vi "Populate File Info.vi"(8 "error in":errorcluster, 11 "UI Actor in":refnum<class "UI Actor.lvclass">) -> (0 "error out":errorcluster, 3 "UI Actor out":refnum<class "UI Actor.lvclass">)   [LabVIEW 2024, in "UI Actor.lvlib" / "UI Actor.lvclass"]
uses:
  UI Actor.lvclass
  Controls/File Info.ctl
  UI Actor.lvclass/UI Actor.ctl
  Core/File Info/File Info.lvclass
  Core/EDS/EDS.lvclass
  <vilib>/Utility/Data Type/NI_Data Type.lvlib
  <userlib>/_OpenG.lib/lvdata/lvdata.llb/openg_variant.lvlib
  <vilib>/JDP Science/JDP Science Common Utilities/JDP Utility.lvlib
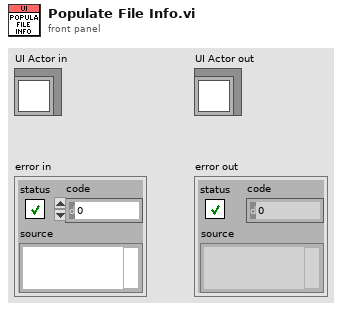
[diagram p1: front panel]
types:
  T1 = typedef "File Info.ctl" = cluster{"FileVersion":u8, "FileRevision":u8, "EDSVersion":string, "Description":string, "CreationDate":string, "CreationTime":string, "CreatedBy":string, "ModificationDate":string, "ModificationTime":string, "ModifiedBy":string}
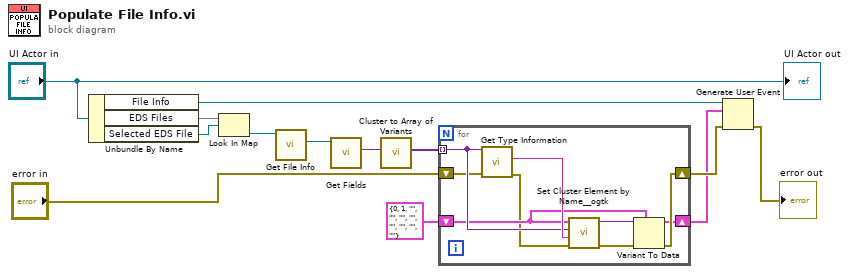
[diagram p0: block diagram]
diagram:
  n1 = Unbundle By Name("UI Actor in") -> ("File Info"=w13:refnum<user-event>, "EDS Files"=w9:map{path, refnum<class "EDS.lvclass">}, "Selected EDS File"=w8:path)
  n2 = Look In Map(map=w9, key=w8) -> (value=w10:refnum<class "EDS.lvclass">)  [unwired: 1 in, 1 out]
  n3 = call "Get File Info.vi"("EDS in"=w10) -> ("File Info"=w5:refnum<class "File Info.lvclass">)  [unwired: 9 in, 1 out]
  n4 = call-dynamic "Get Fields.vi"("File Info in"=w5) -> ("Fields"=w7:variant)  [unwired: 9 in, 1 out]
  n5 = call <vilib>:"Cluster to Array of Variants.vi"("Cluster"=w7) -> ("Array of Cluster Elements"=w6:variant[])  [unwired: 10 in]
  n6 = for {
    tunnel: w6 -> [w21] mode=indexing
    shift-right: [w16] -> w2
    shift-left: T1 {"FileVersion"=0, "FileRevision"=1, "EDSVersion"="", "Description"="", "CreationDate"="", "CreationTime"="", "CreatedBy"="", "ModificationDate"="", "ModificationTime"="", "ModifiedBy"=""} ("EDS File Info") -> [w17]
    shift-right: [w19] -> w3
    shift-left: "error in" -> [w15]
    n7 = call <vilib>:"Get Type Information.vi"("error in (no error)"=w15, "variant"=w21) -> ("error out"=w14:errorcluster, "name"=w22:string)  [unwired: 5 in, 3 out]
    n8 = call <userlib>:"Set Cluster Element by Name__ogtk.vi"("error in (no error)"=w14, "Element Name (\"\": New Element Data Name)"=w22, "New Element Value"=w21, "Cluster"=w17) -> ("error out"=w20:errorcluster, "VCluster out"=w18:variant)  [unwired: 5 in, 1 out]
    n9 = Variant To Data(error in=w20, type=w17, Variant=w18) -> (data=w16:T1, error out=w19:errorcluster)
  }
  n10 = Generate User Event(user event=w13, event data cluster=w2, error in=w3) -> (error out=→"error out":errorcluster)  [unwired: 1 in, 1 out]
  "UI Actor out" <- "UI Actor in"
